vi "Botones Global.vi"() -> ()   [LabVIEW 2014]
panel:
  out "botones":T1
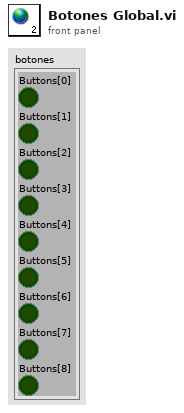
[diagram p1: front panel]
types:
  T1 = cluster{"Buttons[0]":bool, "Buttons[1]":bool, "Buttons[2]":bool, "Buttons[3]":bool, "Buttons[4]":bool, "Buttons[5]":bool, "Buttons[6]":bool, "Buttons[7]":bool, "Buttons[8]":bool}
diagram:
